vi "Decimate Metrics.vi"() -> ()   [LabVIEW 2019]
panel:
  out "Decimation Factor":i32
  out "Fs":dbl
  out "Waveform Graph":waveform(dbl)[](graph)
  out "XY Graph 5":cluster{i32[], dbl[]}[](graph)=[{[2048, 2001, 1955, 1911, 1867, 1825, 1783, 1743, 1703, 1664, 1626, 1589, 1553, 1518, 1483, 1449, 1416, 1384, 1353, 1322, 1292, 1262, 1234, 1205, 1178, 1151, 1125, 1099, 1074, 1050, 1026, 1003, 980, 957, 936, 914, 893, 873, 853, 834, 815, 796, 778, 760, 743, 726, 710, 693, 678, 662, 647, 632, 618, 604, 590, 577, 564, 551, 538, 526, 514, 502, 491, 480, 469, 458, 448, 437, 427, 418, 408, 399, 390, 381, 372, 364, 355, 347, 339, 332, 324, 317, 309, 302, 296, 289, 282, 276, 269, 263, 257, 251, 246, 240, 235, 229, 224, 219, 214, 209, 204, 200, 195, 191, 186, 182, 178, 174, 170, 166, 162, 158, 155, 151, 148, 144, 141, 138, 135, 132, 129, 126, 123, 120, 117, 115, 112, 109, 107, 105, 102, 100, 98, 95, 93, 91, 89, 87, 85, 83, 81, 79, 77, 76, 74, 72, 71, 69, 67, 66, 64, 63, 61, 60, 59, 57, 56, 55, 53, 52, 51, 50, 49, 48, 46, 45, 44, 43, 42, 41, 40, 39, 39, 38, 37, 36, 35, 34, 33, 33, 32, 31, 30, 30, 29, 28, 28, 27, 26, 26, 25, 25, 24, 24, 23, 22, 22, 21, 21, 20, 20, 20, 19, 19, 18, 18, 17, 17, 17, 16, 16, 15, 15, 15, 14, 14, 14, 13, 13, 13, 12, 12, 12, 12, 11, 11, 11, 10, 10, 10, 10, 10, 9, 9, 9, 9, 8, 8, 8, 8, 8, 7, 7, 7, 7, 7, 7, 6, 6, 6, 6, 6, 6, 6, 5, 5, 5, 5, 5, 5, 5, 5, 4, 4, 4, 4, 4, 4, 4, 4, 4, 3, 3, 3, 3, 3, 3, 3, 3, 3, 3, 3, 3, 3, 2, 2, 2, 2, 2, 2, 2, 2, 2, 2, 2, 2, 2, 2, 2, 2, 2, 2, 1, 1, 1, 1, 1, 1, 1, 1, 1], [9.456700034206733e-06, 1.4248999126721173e-05, 9.65880005969666e-06, 9.584400017047301e-06, 1.5311900206143037e-05, 9.544799861032516e-06, 9.621600358514114e-06, 9.617400268325583e-06, 9.648200211813674e-06, 9.583599632605911e-06, 9.525099972961471e-06, 9.602400357834994e-06, 9.67980016139336e-06, 9.78039944311604e-06, 1.5311299997847527e-05, 1.540020015090704e-05, 9.776199498446658e-06, 9.713500185171143e-06, 9.738200315041468e-06, 9.686899633379653e-06, 1.5308600093703715e-05, 9.584099490894005e-06, 9.592300426447765e-06, 9.65300021925941e-06, 9.635300317313522e-06, 9.518000559182838e-06, 9.556000062730164e-06, 9.558999649016187e-06, 1.530009930138476e-05, 9.566000488121062e-06, 9.600599354598671e-06, 9.70719987526536e-06, 9.678600152255967e-06, 9.704799624159932e-06, 9.698599838884547e-06, 1.5491100784856827e-05, 9.845199791016057e-06, 9.806500311242416e-06, 9.797699865885078e-06, 9.85189972561784e-06, 9.87670005997643e-06, 9.740100387716665e-06, 1.5268799994373694e-05, 1.0015301377279684e-05, 1.6252900415565817e-05, 1.5496199805056678e-05, 1.0026199597632512e-05, 1.0094099387060851e-05, 1.0099700099090115e-05, 1.5573800395941363e-05, 1.5630600188160315e-05, 9.755000355653465e-06, 9.65000013820827e-06, 1.5413200104376302e-05, 1.0095400095451623e-05, 9.845299646258354e-06, 9.779300424270333e-06, 9.770900098374113e-06, 1.5396900242194534e-05, 1.5296499303076417e-05, 1.5401999640744178e-05, 9.630500135244802e-06, 9.732600126881152e-06, 1.542950014118105e-05, 9.835899691097438e-06, 9.842799918260426e-06, 1.554069947451353e-05, 1.5411400236189367e-05, 1.5389499807497487e-05, 9.641999669838697e-06, 9.889800450764597e-06, 9.872500086203218e-06, 9.842298983130605e-06, 9.869499452179298e-06, 9.91939994855784e-06, 9.816500067245215e-06, 9.826799971051515e-06, 9.76220049778931e-06, 1.5495500265387817e-05, 1.548109992290847e-05, 1.553970025270246e-05, 1.0033599828602746e-05, 1.0059700493002311e-05, 1.5636999829439446e-05, 9.859400597633794e-06, 1.5501699992455543e-05, 1.6100100125186145e-05, 1.0024899762356654e-05, 1.6049499390646815e-05, 1.011679955990985e-05, 1.5650800109142437e-05, 1.0113899654243141e-05, 1.6021600080421193e-05, 1.0137800156371669e-05, 1.5795499755768104e-05, 1.583949933410622e-05, 1.0043800517451018e-05, 1.0094100551214069e-05, 1.0051999968709424e-05, 1.0049600212369115e-05, 9.979500668123365e-06, 1.004489991464652e-05, 9.980599628761411e-06, 1.544610023847781e-05, 1.0343399801058695e-05, 1.014409982599318e-05, 1.0266698780469596e-05, 1.0084300127346068e-05, 1.0002600407460705e-05, 1.57064993691165e-05, 1.5843399829464033e-05, 0.011003955555174293, 0.011012422221635157, 0.01087487777759735, 0.010866200001651628, 0.010824011118125377, 0.010891299998749875, 0.010893677775230672, 0.010829544445085857, 0.011031377776008513, 0.011514344440203987, 0.011566433331204785, 0.011276411115735149, 0.011790412496338831, 0.011058433337085363, 0.011251366671381725, 0.011618211111959277, 0.011475344447212087, 0.011457166666837616, 0.011109844448381208, 0.011006822221032862, 0.010873122221609164, 0.010887122218264267, 0.010909477782358104, 0.01103178888378251, 0.010794266667087667, 0.010844022229624292, 0.01144321111173162, 0.01094655555465983, 0.010804177779290412, 0.011677544441125873, 0.010860166661182625, 0.010990366669526944, 0.010932444442813802, 0.010868422218158634, 0.01084767778067746, 0.011066922222703902, 0.011144555548930334, 0.011144844440018965, 0.010890188885645734, 0.010836322219499076, 0.011004333332594898, 0.010930555555710776, 0.011527433331745366, 0.010895133328934511, 0.011756344452603824, 0.011065488894625256, 0.011515822219533019, 0.011476711108116433, 0.010889399990749856, 0.01094971111160703, 0.01090683333718011, 0.010953755564211557, 0.010859822227050446, 0.010934077772415347, 0.011478888896009367, 0.010827400000481349, 0.010831433335422642, 0.010872866664107682, 0.01084597777420034, 0.011458577772524828, 0.010886666668941163, 0.010878633342347004, 0.010823677779020121, 0.011056733333842002, 0.010938366664858121, 0.010830522223841399, 0.010821911108602459, 0.010851633334014978, 0.01081431110893997, 0.010836455557081435, 0.010990722218088599, 0.010906577776444869, 0.011522377779733183, 0.010832866666735046, 0.011494444443896, 0.010861666669370607, 0.011007622223890698, 0.010963211110922404, 0.011448499998853853, 0.010877633331498751, 0.010913277775721831, 0.01093590000204535, 0.01079776667433584, 0.011499088888134187, 0.011405866667498939, 0.01143516666100671, 0.010840033332998347, 0.012053599991809784, 0.011425122220922882, 0.011014722222979698, 0.012736962497001514, 0.011027000000467524, 0.01119901111168373, 0.011394588887924328, 0.011256511109725883, 0.011025455550730435, 0.01136748888853213, 0.01108531111256323, 0.011000499992708987, 0.011047344441370418, 0.01108172222221684, 0.011061599995527003, 0.010961288890232228, 0.011215044440986175, 0.011114766666044792, 0.011719299997720454, 0.011080477777997859, 0.011952300003031269, 0.011660300004425354, 0.011049588893203892, 0.01167258888664138, 0.011830488882777799, 0.01106242222401003, 0.011723633331712335, 0.011531033326819953, 0.01094046666791352, 0.010917111109140225, 0.011036200002611926, 0.011082066666050296, 0.010971955550808666, 0.010912011109111417, 0.010944677775518762, 0.011557333333055593, 0.011587944444424162, 0.010973933330711184, 0.010967644435974458, 0.011541144440545596, 0.010871100003391298, 0.010831466662542274, 0.011458311113528907, 0.010914799999833727, 0.011838022215265987, 0.011006799998641428, 0.010897599994981041, 0.010892722215632804, 0.010925255550925309, 0.01085896666498027, 0.01147336666407581, 0.010934688884946, 0.010880411111025346, 0.01085462222302643, 0.011402688888160305, 0.010853555561172672, 0.011497444444103166, 0.010839466668484319, 0.011423655559257086, 0.010828277775241682, 0.010844077782369115, 0.011558422223768301, 0.010887800007670497, 0.010836944443225447, 0.010942299999037964, 0.010927011113381013, 0.010997677774867043, 0.011424255547656989, 0.010846555556377603, 0.010884111110095141, 0.011532966668407122, 0.010866044438444078, 0.010832844441109855, 0.01087096666257518, 0.010868622219681533, 0.010944899996199334, 0.010899588889313035, 0.010870755556324083, 0.011110688883086873, 0.011010322225047275, 0.011428511109746372, 0.010866399999940768, 0.011504155561043363, 0.010903688888194867, 0.010936755547946733, 0.01081154445031037, 0.010847233329615038, 0.012186012503661914, 0.012253487500856863, 0.012488625001424225, 0.01320933749593678, 0.012182649999886053, 0.012187400003313087, 0.012167937500635162, 0.0121895999982371, 0.012263612494280096, 0.013132212494383566, 0.012205300005007302, 0.012179512501461431, 0.012254712499270681, 0.012818837501981761, 0.012290562499401858, 0.012927650001074653, 0.012167587501608068, 1.4772199850995094e-05, 1.4771599875530227e-05, 1.4787899912334978e-05, 1.4792299974942579e-05, 1.5060800011269748e-05, 1.4905399846611545e-05, 1.4904899609973654e-05, 1.4919400069629774e-05, 1.4973499986808748e-05]}, ...(3 in all)]
  out "XY Graph 4":cluster{"Fs":dbl[], dbl[]}[](graph)
  out "XY Graph 3":cluster{dbl[], dbl[]}(graph)={[170.0, 170.0, 170.0, 170.0, 170.0, 169.0, 169.0, 169.0, 169.0, 169.0, 169.0, 169.0, 168.0, 168.0, 168.0, 168.0, 168.0, 168.0, 168.0, 168.0, 167.0, 167.0, 167.0, 167.0, 167.0, 167.0, 167.0, 166.0, 166.0, 166.0, 166.0, 166.0, 166.0, 166.0, 165.0, 165.0, 165.0, 165.0, 165.0, 165.0, 165.0, 165.0, 164.0, 164.0, 164.0, 164.0, 164.0, 164.0, 164.0, 163.0, 163.0, 163.0, 163.0, 163.0, 163.0, 163.0, 163.0, 162.0, 162.0, 162.0, 162.0, 162.0, 162.0, 162.0, 162.0, 161.0, 161.0, 161.0, 161.0, 161.0, 161.0, 161.0, 161.0, 160.0, 160.0, 160.0, 160.0, 160.0, 160.0, 160.0, 160.0, 159.0, 159.0, 159.0, 159.0, 159.0, 159.0, 159.0, 159.0, 158.0, 158.0, 158.0, 158.0, 158.0, 158.0, 158.0, 158.0, 157.0, 157.0, 157.0, 157.0], [4.5953500230098146e-05, 4.542210011277348e-05, 4.5567599765490743e-05, 4.903029976412654e-05, 5.188759951852262e-05, 4.657020000740886e-05, 4.474290058715269e-05, 4.478939960245043e-05, 4.4684299820801244e-05, 4.5100099901901556e-05, 4.518199959420599e-05, 4.495499999029562e-05, 4.487900051753968e-05, 4.507460023160092e-05, 4.482510028174147e-05, 4.505990011966787e-05, 4.508440018980764e-05, 4.533870014711283e-05, 4.516969929682091e-05, 4.501400038134307e-05, 4.5748500415356827e-05, 4.5786499715177344e-05, 4.602679974050261e-05, 4.579390009166673e-05, 4.5730299490969626e-05, 4.549530043732375e-05, 4.539970055338927e-05, 4.448479987331666e-05, 4.4368800532538445e-05, 4.468309972435236e-05, 4.459529955056496e-05, 4.497959997388534e-05, 4.478320060297847e-05, 4.522879995056428e-05, 4.58569998445455e-05, 4.6199699689168484e-05, 4.599359969142824e-05, 4.606779984897003e-05, 4.5954200613778086e-05, 4.592010003398172e-05, 4.6736499964026737e-05, 4.6116199751850216e-05, 4.6079799445578825e-05, 4.581690009217709e-05, 4.575130032026209e-05, 4.5685000251978635e-05, 4.5807799993781374e-05, 4.590420000022277e-05, 4.6118599886540326e-05, 4.5160400040913374e-05, 4.48098998167552e-05, 4.459749968373217e-05, 4.463830037275329e-05, 4.4440799683798105e-05, 4.5866699423640963e-05, 4.443210078170523e-05, 4.482760024257004e-05, 4.691510045086034e-05, 4.721850046189502e-05, 4.6634400117909536e-05, 4.677460002130829e-05, 4.6209200634621084e-05, 4.6702099614776674e-05, 4.643399981432594e-05, 4.627189983148128e-05, 4.478789929999039e-05, 4.565320062101819e-05, 4.49053005722817e-05, 4.484229965601116e-05, 4.470609975396656e-05, 4.4670200091786684e-05, 4.4783400313463064e-05, 4.486910047126003e-05, 0.0874482500027322, 0.08829841666738503, 0.08722880000035123, 0.08717403333381905, 0.08697311666522485, 0.08667569998942781, 0.086163783329539, 0.08643608333174295, 0.08734118333571435, 0.08763096666370984, 0.08779845000147664, 0.08668426666311764, 0.08676534999782841, 0.08764381667424459, 0.08733363334128323, 0.08726173333222202, 0.0874043000076199, 0.08637073333375156, 0.08583501666241015, 0.08690373333714281, 0.08906938333529979, 0.08884371666742179, 0.08933958334576649, 0.08936326666541088, 0.0876478833379224, 0.08779091665928718, 0.08782516666785038, 0.08712571665819269]}
  out "XY Graph 2":cluster{"Fs":dbl[], dbl[]}[](graph)=[{"Fs"=[1200.0, 1201.0, 1202.0, 1203.0, 1204.0, 1205.0, 1206.0, 1207.0, 1208.0, 1209.0, 1210.0, 1211.0, 1212.0, 1213.0, 1214.0, 1215.0, 1216.0, 1217.0, 1218.0, 1219.0, 1220.0, 1221.0, 1222.0, 1223.0, 1224.0, 1225.0, 1226.0, 1227.0, 1228.0, 1229.0, 1230.0, 1231.0, 1232.0, 1233.0, 1234.0, 1235.0, 1236.0, 1237.0, 1238.0, 1239.0, 1240.0, 1241.0, 1242.0, 1243.0, 1244.0, 1245.0, 1246.0, 1247.0, 1248.0, 1249.0, 1250.0, 1251.0, 1252.0, 1253.0, 1254.0, 1255.0, 1256.0, 1257.0, 1258.0, 1259.0, 1260.0, 1261.0, 1262.0, 1263.0, 1264.0, 1265.0, 1266.0, 1267.0, 1268.0, 1269.0, 1270.0, 1271.0, 1272.0, 1273.0, 1274.0, 1275.0, 1276.0, 1277.0, 1278.0, 1279.0, 1280.0, 1281.0, 1282.0, 1283.0, 1284.0, 1285.0, 1286.0, 1287.0, 1288.0, 1289.0, 1290.0, 1291.0, 1292.0, 1293.0, 1294.0, 1295.0, 1296.0, 1297.0, 1298.0, 1299.0, 1300.0], [4.5953500230098146e-05, 4.542210011277348e-05, 4.5567599765490743e-05, 4.903029976412654e-05, 5.188759951852262e-05, 4.657020000740886e-05, 4.474290058715269e-05, 4.478939960245043e-05, 4.4684299820801244e-05, 4.5100099901901556e-05, 4.518199959420599e-05, 4.495499999029562e-05, 4.487900051753968e-05, 4.507460023160092e-05, 4.482510028174147e-05, 4.505990011966787e-05, 4.508440018980764e-05, 4.533870014711283e-05, 4.516969929682091e-05, 4.501400038134307e-05, 4.5748500415356827e-05, 4.5786499715177344e-05, 4.602679974050261e-05, 4.579390009166673e-05, 4.5730299490969626e-05, 4.549530043732375e-05, 4.539970055338927e-05, 4.448479987331666e-05, 4.4368800532538445e-05, 4.468309972435236e-05, 4.459529955056496e-05, 4.497959997388534e-05, 4.478320060297847e-05, 4.522879995056428e-05, 4.58569998445455e-05, 4.6199699689168484e-05, 4.599359969142824e-05, 4.606779984897003e-05, 4.5954200613778086e-05, 4.592010003398172e-05, 4.6736499964026737e-05, 4.6116199751850216e-05, 4.6079799445578825e-05, 4.581690009217709e-05, 4.575130032026209e-05, 4.5685000251978635e-05, 4.5807799993781374e-05, 4.590420000022277e-05, 4.6118599886540326e-05, 4.5160400040913374e-05, 4.48098998167552e-05, 4.459749968373217e-05, 4.463830037275329e-05, 4.4440799683798105e-05, 4.5866699423640963e-05, 4.443210078170523e-05, 4.482760024257004e-05, 4.691510045086034e-05, 4.721850046189502e-05, 4.6634400117909536e-05, 4.677460002130829e-05, 4.6209200634621084e-05, 4.6702099614776674e-05, 4.643399981432594e-05, 4.627189983148128e-05, 4.478789929999039e-05, 4.565320062101819e-05, 4.49053005722817e-05, 4.484229965601116e-05, 4.470609975396656e-05, 4.4670200091786684e-05, 4.4783400313463064e-05, 4.486910047126003e-05, 0.0874482500027322, 0.08829841666738503, 0.08722880000035123, 0.08717403333381905, 0.08697311666522485, 0.08667569998942781, 0.086163783329539, 0.08643608333174295, 0.08734118333571435, 0.08763096666370984, 0.08779845000147664, 0.08668426666311764, 0.08676534999782841, 0.08764381667424459, 0.08733363334128323, 0.08726173333222202, 0.0874043000076199, 0.08637073333375156, 0.08583501666241015, 0.08690373333714281, 0.08906938333529979, 0.08884371666742179, 0.08933958334576649, 0.08936326666541088, 0.0876478833379224, 0.08779091665928718, 0.08782516666785038, 0.08712571665819269]}]
  out "XY Graph":cluster{"Fs":dbl[], dbl[]}[](graph)=[{"Fs"=[10.0, 11.220184543019636, 12.589254117941675, 14.12537544622754, 15.848931924611133, 17.78279410038923, 19.952623149688797, 22.3872113856834, 25.118864315095795, 28.183829312644534, 31.622776601683793, 35.48133892335755, 39.810717055349734, 44.6683592150963, 50.11872336272725, 56.23413251903491, 63.09573444801933, 70.79457843841381, 79.43282347242814, 89.12509381337459, 100.0, 112.2018454301963, 125.89254117941675, 141.25375446227554, 158.48931924611142, 177.82794100389228, 199.52623149688787, 223.872113856834, 251.18864315095823, 281.8382931264455, 316.22776601683796, 354.8133892335753, 398.1071705534973, 446.6835921509635, 501.18723362727246, 562.341325190349, 630.957344480193, 707.945784384138, 794.3282347242822, 891.2509381337459, 1000.0, 1122.018454301964, 1258.9254117941675, 1412.537544622754, 1584.893192461114, 1778.2794100389228, 1995.262314968881, 2238.72113856834, 2511.886431509582, 2818.382931264455, 3162.2776601683795], [3.607890009880066e-05, 3.764839968062006e-05, 3.577880054945126e-05, 3.603930061217397e-05, 3.629109999747015e-05, 3.932959985104389e-05, 3.9221000246470795e-05, 3.923630045028403e-05, 3.962909954134375e-05, 3.920570039190352e-05, 3.8993100490188224e-05, 3.927989979274571e-05, 3.358929944806732e-05, 3.387029969599098e-05, 3.3943500340683385e-05, 3.390460013179108e-05, 3.389760089339689e-05, 3.37506000942085e-05, 3.420749958604574e-05, 3.3667800133116543e-05, 3.3919001056347045e-05, 3.367859977879562e-05, 3.41453998698853e-05, 3.4131499793147666e-05, 3.3739300240995365e-05, 3.3986599650233985e-05, 3.4082300262525676e-05, 3.4326000342844056e-05, 3.47152998438105e-05, 3.5184600274078546e-05, 3.859700020984746e-05, 3.8918899983400476e-05, 3.893959990818985e-05, 3.864399995654821e-05, 3.9217499899677935e-05, 3.873230001772754e-05, 3.9916600479045883e-05, 4.0908599621616305e-05, 4.088079967186786e-05, 4.11779002752155e-05, 4.199039968079888e-05, 4.297219958971254e-05, 4.261799974483438e-05, 0.08745993332316478, 0.08677018332916002, 0.08683001667183514, 0.08679753332398832, 0.08593768333957996, 0.08655301665809627, 0.08669649999743949, 0.0876208833263566]}, {"Fs"=[10.0, 11.220184543019636, 12.589254117941675, 14.12537544622754, 15.848931924611133, 17.78279410038923, 19.952623149688797, 22.3872113856834, 25.118864315095795, 28.183829312644534, 31.622776601683793, 35.48133892335755, 39.810717055349734, 44.6683592150963, 50.11872336272725, 56.23413251903491, 63.09573444801933, 70.79457843841381, 79.43282347242814, 89.12509381337459, 100.0, 112.2018454301963, 125.89254117941675, 141.25375446227554, 158.48931924611142, 177.82794100389228, 199.52623149688787, 223.872113856834, 251.18864315095823, 281.8382931264455, 316.22776601683796, 354.8133892335753, 398.1071705534973, 446.6835921509635, 501.18723362727246, 562.341325190349, 630.957344480193, 707.945784384138, 794.3282347242822, 891.2509381337459, 1000.0, 1122.018454301964, 1258.9254117941675, 1412.537544622754, 1584.893192461114, 1778.2794100389228, 1995.262314968881, 2238.72113856834, 2511.886431509582, 2818.382931264455, 3162.2776601683795], [0.0875007999954202, 0.0868551666693141, 0.00011527660037972964, 5.173529972671531e-05, 0.08731953334063292, 6.382310003391467e-05, 5.987870047101751e-05, 6.096380067174323e-05, 5.121290049282834e-05, 5.942010035505518e-05, 5.7633300428278746e-05, 0.08728604999487288, 5.1549999916460365e-05, 5.689030018402264e-05, 5.27350994234439e-05, 4.455230029998347e-05, 0.08695533333714896, 5.2730599883943794e-05, 4.736569954548031e-05, 4.719190017203801e-05, 0.1742585000077573, 0.08824173332929301, 5.0185800151666626e-05, 0.08803653333840582, 0.08699571666268942, 4.2394200136186555e-05, 0.08714776667087183, 4.5517299993662166e-05, 4.5455199433490634e-05, 0.0879902166731578, 4.443929970148019e-05, 4.4665599998552354e-05, 4.8483799706446005e-05, 4.936830050428398e-05, 0.08728113333927467, 0.08639446666832858, 0.08720138333834863, 0.08710741666436661, 4.46554999507498e-05, 4.5357599185081197e-05, 0.08738301667229582, 0.08707503333183315, 0.08770193333233085, 0.08752203332066226, 0.08630306666600518, 0.08737004999905669, 0.08703096665946457, 0.08639635000145063, 0.08640141666789229, 0.08778989999458038, 0.17497280000437362]}]
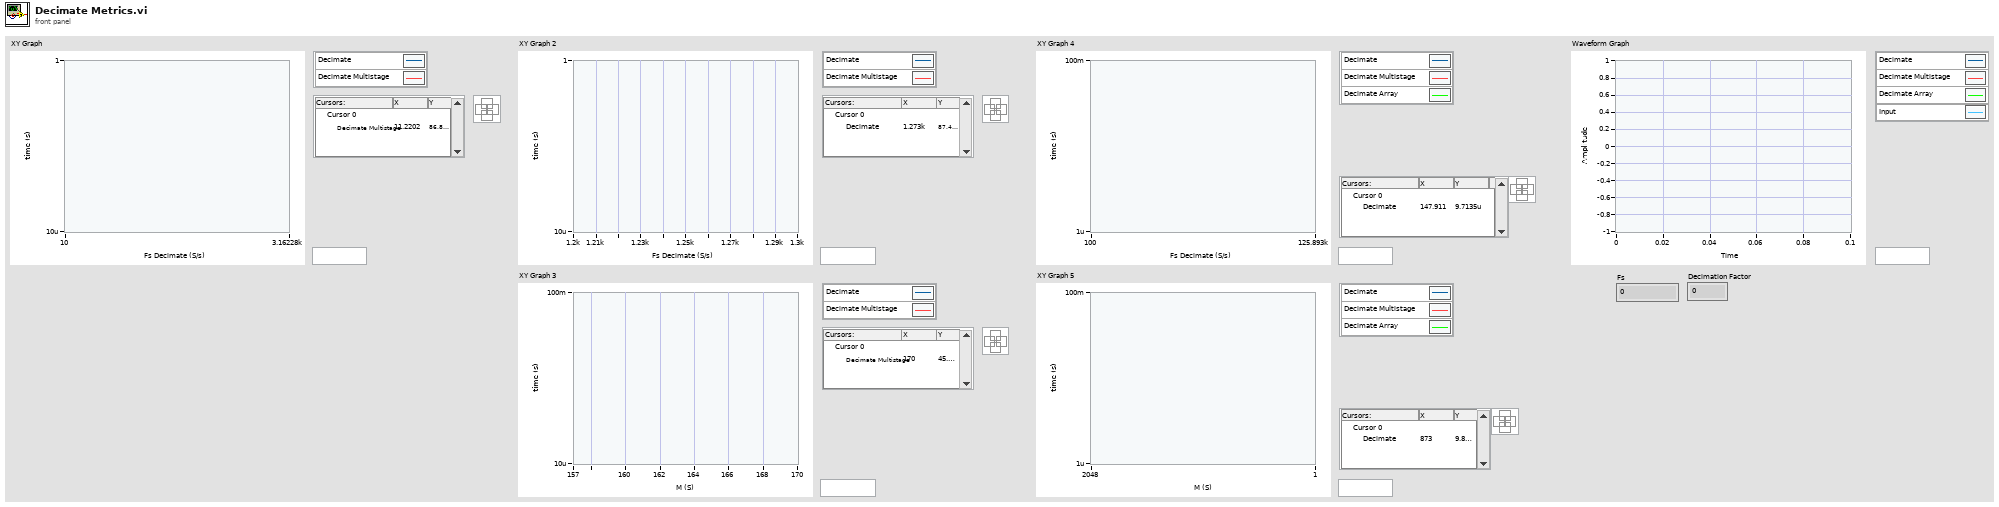
[diagram p1: front panel]
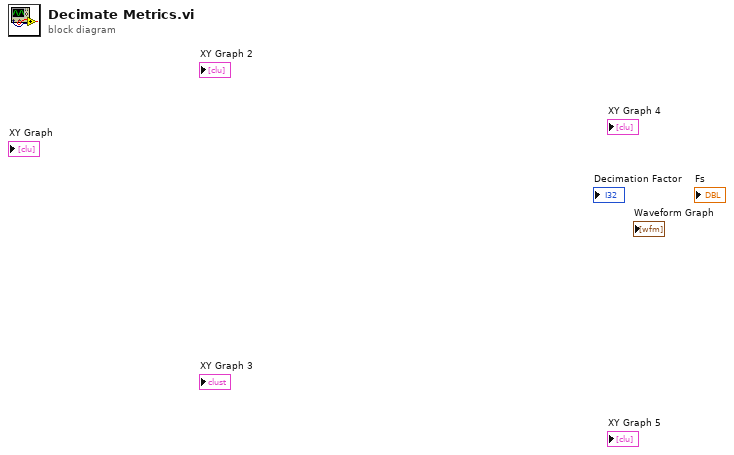
[diagram p0: block diagram]
diagram:
